vi "GL_Rapid_Scan_Trigs.vi"(0 "GL Ref Out":refnum<k7>, 1 "Program Name":string caption="Beginning Text", 2 "Start Position":i32=500000, 3 "BKPT Shift":i32, 5 "Axis":i32, 7 "Pause?":bool, 9 "# frames/ s":sgl, 11 "error in":errorcluster, 12 "overshoot":i32=500, 13 "step interval":i32, 14 "Total Steps (one way)":i32) -> (4 "ref out":refnum<k7>, 6 "Axis Out":i32, 15 "error out":errorcluster)   [LabVIEW 2022 SP3]
doc: "EXAMPLE: DO_WHILE Loop (Onboard Programming Template)\n\nSUMMARY:\nThis FlexMotion example demonstrates the implementation of a DO_WHILE loop data structure in an onboard program. The C equivalent of the data structure implemented here is:\n\ndo {\n// code to be repeated\nloopVar = loopVar - increment;\n} while (loopVar != 0);\n\nTHEORY OF OPERATION:\nThe flow of the DO_WHILE loop data structure goes as follows:\n(1) Program storage is begun.\n(2) The DO_WHILE loop is set up. (Loop Variable and Increment are each defined and initialized.)\n(3) A code delimiter is set using label #1.\n(4) Code to be executed each time through loop is run (in the template program, the loop variable is decremented).\n(5) The loop variable or other test condition is checked.\n(6) If the test condition is true, then we jump back to label #1. Otherwise, the condition is false so the loop terminates.\n(7) Program storage is ended.\n\nDEVELOPMENT DETAILS:\nApplication Software: LabVIEW 5.0.x\nHardware: FlexMotion controller\nDriver Software: FlexMotion Software 4.0\n\nREQUIRED HARDWARE:\n(controller only)\n\nINSTRUCTIONS:\n(0) Initialize the FlexMotion controller before running this VI. \n(1) Add the FlexMotion functions you want to execute into the block diagram where noted.\n(2) Run the VI to store the program. (The program will not be executed at this time.)\n(3) You can then run the program you have stored by calling the run_prog.flx function with the appropriate program number.\n\nADDITIONAL NOTES:\n(a) You should read the following items before writing FlexMotion onboard programs:\n(1) The Onboard Programs section of the FlexMotion Hardware User Manual (page 4-9 in the November 1998 edition).\n(2) The section about onboard variables in your FlexMotion Software Reference Manual (pages 4-11 and 4-12 in the November 1998 edition)\n(3) You will find the chapter of the FlexMotion Software Reference Manual concerning the Onboard Programming functions to be an invaluable reference resource (Chapter 12 of the November 1998 edition) along with the online help for the VI functions.\n(b) This template repeats the DO_WHILE loop as long as an expression with a variable evaluates to be true. However, you may evaluate other conditions such as move complete status instead.\n\n*NOTE: This example is not supported on the 7334 controller."
panel:
  out "acc (mm/s^2)":dbl
  out "velocity (mm/s)":dbl=10000.0
  out "1st BKPT":i32
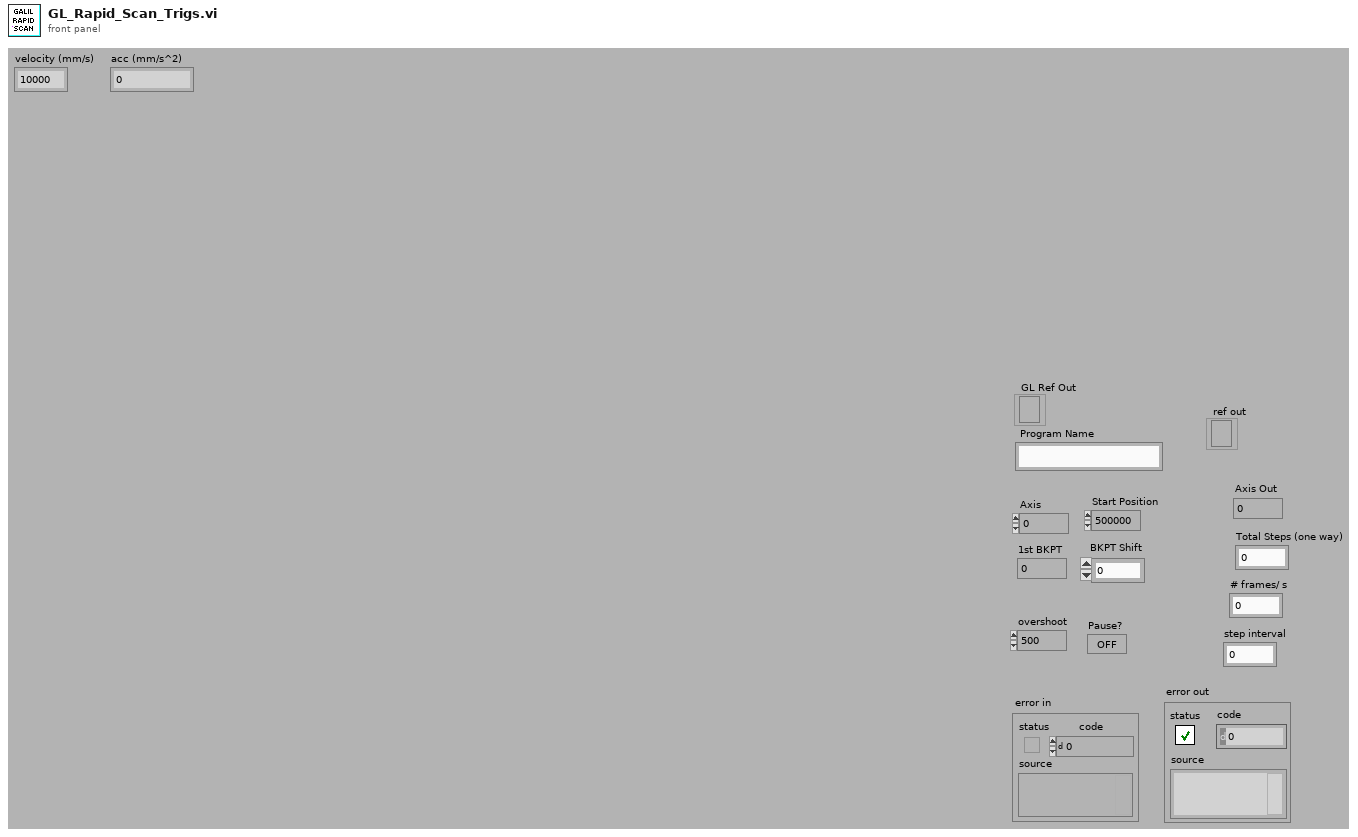
[diagram p1: front panel]
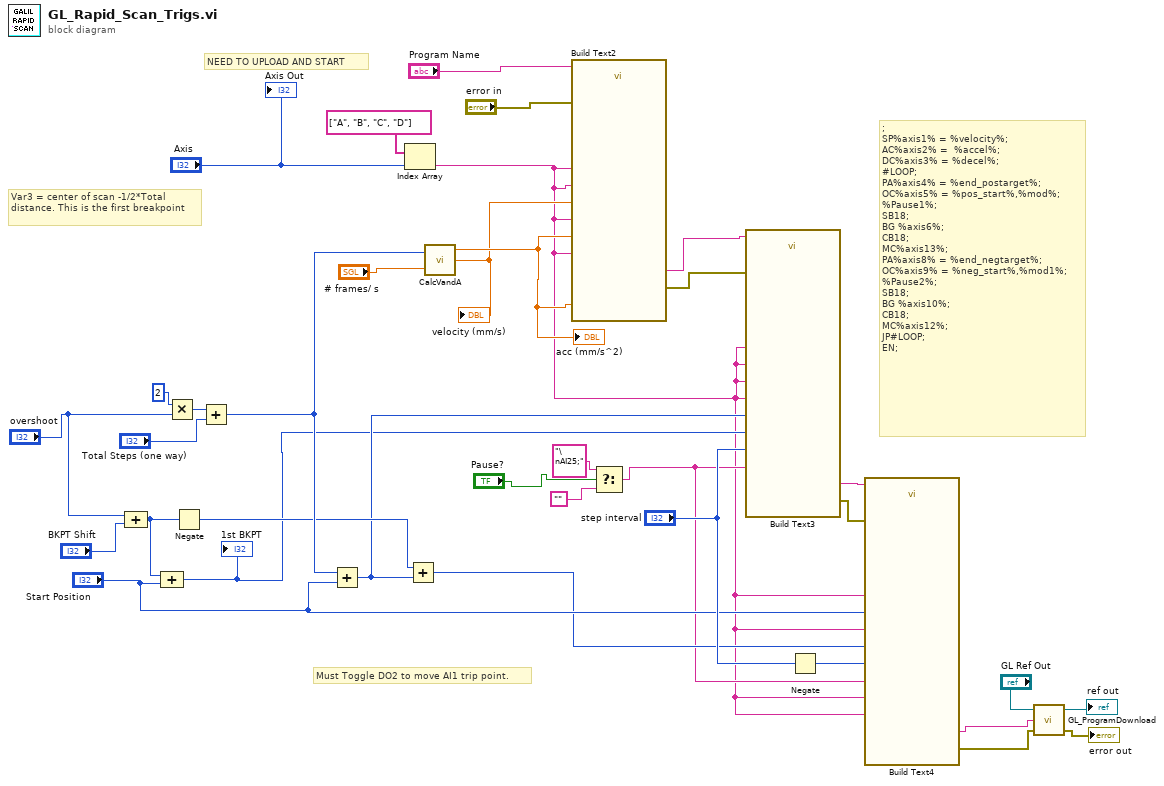
[diagram p0: block diagram]
diagram:
  # "Must Toggle DO2 to move AI1 trip point."
  # "NEED TO UPLOAD AND START"
  # ";\nSP%axis1% = %velocity%;\nAC%axis2% =  %accel%;\nDC%axis3% = %decel%;\n#LOOP;\nPA%axis4% = %end_postarget%;\nOC%axis5% = %pos_start%,%mod%;\n%Pause1%;\nSB18;\nBG %axis6%;\nCB18;\nMC%axis13%;\nPA%axis8% = %end_negtarget%;\nOC%axis9% = %neg_start%,%mod1%;\n%Pause2%;\nSB18;\nBG %axis10%;\nCB18;\nMC%axis12%;\nJP#LOOP;\nEN;"
  # "Var3 = center of scan -1/2*Total distance. This is the first breakpoint"
  n1 = Compound Arithmetic op=ADD("overshoot", "BKPT Shift") -> (w31:i32)
  n2 = Compound Arithmetic op=ADD(w31, "Start Position") -> (w20:i32)
  "1st BKPT" <- w20
  n3 = Multiply(x=2, y="overshoot") -> (x*y=w34:i32)
  n4 = Negate(x=w31) -> (-x=w23:i32)
  n5 = Add(x=w34, y="Total Steps (one way)") -> (x+y=w33:i32)
  n6 = Add(x=w33, y="Start Position") -> (x+y=w21:i32)
  n7 = Index Array(array=string[] ["A", "B", "C", "D"], index="Axis") -> (element=w1:string)
  n8 = Add(x=w23, y=w21) -> (x+y=w16:i32)
  n9 = call "CalcVandA.vi"("distance"=w33, "fps"="# frames/ s") -> ("Accel"=w3:dbl, "Velocity"=w2:dbl)  [unwired: 1 out]
  "velocity (mm/s)" <- w2
  "acc (mm/s^2)" <- w3
  n10 = call "Build Text2"("Beginning Text"="Program Name", "axis2"=w1, "axis3"=w1, "axis1A"=w1, "axis1"=w1, "velocity"=w2, "error in (no error)"="error in", "accel"=w3, "decel"=w3) -> ("Result"=w11:string, "error out"=w12:errorcluster)  [unwired: 5 in]
  n11 = Select(t="\nAI25;", s="Pause?", f="") -> (s? t:f=w14:string)
  n12 = call "Build Text3"("Beginning Text"=w11, "pos_start"=w20, "Pause1"=w14, "axis13"=w1, "axis4"=w1, "end_postarget"=w21, "axis5"=w1, "error in (no error)"=w12, "mod"="step interval", "axis6"=w1) -> ("Result"=w18:string, "error out"=w13:errorcluster)  [unwired: 4 in]
  n13 = Negate(x="step interval") -> (-x=w15:i32)
  n14 = call "Build Text4"("Beginning Text"=w18, "neg_start"=w16, "Pause2"=w14, "axis12"=w1, "axis8"=w1, "end_negtarget"="Start Position", "axis9"=w1, "error in (no error)"=w13, "mod1"=w15, "axis10"=w1) -> ("Result"=w10:string, "error out"=w7:errorcluster)  [unwired: 4 in]
  n15 = call "GL_ProgramDownload.vi"("error in"=w7, "program"=w10, "Galil.IGalil"="GL Ref Out") -> ("error out"=→"error out":errorcluster, "reference out"=→"ref out":refnum<k7>)  [unwired: 1 out]
  "Axis Out" <- "Axis"
